vi "Teleop.vi"(10 "Match Info":T1={"Autonomous Elapsed Seconds"=0.0, "TeleOp Elapsed Seconds"=0.0, "Disabled Elapsed Seconds"=0.0, "Visited Autonomous"=FALSE, "Visited TeleOp"=FALSE, "Visited Disabled"=FALSE, "Autonomous Settings"={"Autonomous Style"=enum."Independent", "VI Refnum"=refnum}}, 11 "Call Context":T2) -> ()   [LabVIEW 2014]
doc: "This VI is called for each TeleOp packet received from the DS where the robot is not disabled. It is often used to read from the joysticks and update I/O or to update setpoints for timed control loops. It should complete and return within 20 milliseconds or it may miss DS packets."
uses:
  Robot Global Data.vi
  <vilib>/functionblocks/FB Core/FB Core.xnode
  <vilib>/functionblocks/Edge Detection/Edge Detect/Edge Detect.vi
  <vilib>/functionblocks/NI_FunctionBlock Libraries.lvlib
  <vilib>/Rock Robotics/WPI/Relay/WPI_RelayValue.ctl
  <vilib>/Rock Robotics/WPI/RobotDrive/WPI_RobotDriveMecanumDrive_Cartesian.vi
  <vilib>/Rock Robotics/WPI/DriverStation/WPI_DriverStationMatch Info.ctl
  <vilib>/Rock Robotics/WPI/DriverStation/WPI_DriverStationDerivedRobotMode.ctl
panel:
  out "One Driver":bool
  out "Loader Up":bool
  out "Right Bumper":bool
  out "Left Bumper":bool
  out "Loader Out":bool
  out "Ejector":bool
  out "Trigger":bool
  out "1 Cylinder":bool
  out "2 Cylinder":bool
  out "3 Cylinder":bool
  out "Motor Values":dbl[](array[numeric])
  out "Gyro Mode?":bool
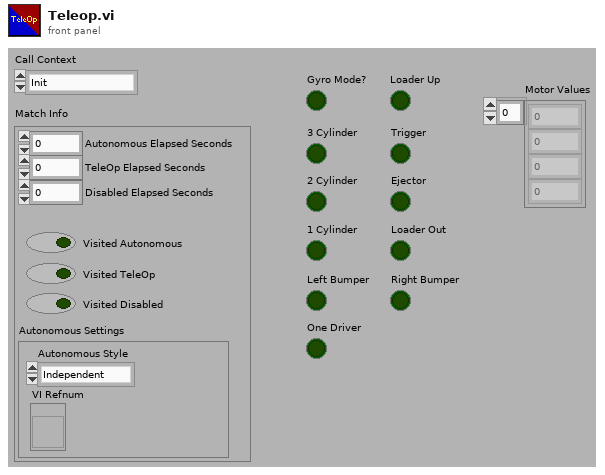
[diagram p1: front panel]
types:
  T1 = typedef "WPI_DriverStationMatch Info.ctl" = cluster{"Autonomous Elapsed Seconds":dbl, "TeleOp Elapsed Seconds":dbl, "Disabled Elapsed Seconds":dbl, "Visited Autonomous":bool, "Visited TeleOp":bool, "Visited Disabled":bool, "Autonomous Settings":cluster{"Autonomous Style":enum16{"Iterative", "Independent"}, "VI Refnum":refnum<vi>}}
  T2 = typedef "WPI_DriverStationDerivedRobotMode.ctl" = enum16{"Init", "Execute", "Stop"}
  T3 = typedef "WPI_RelayValue.ctl" = enum16{"Off", "On", "Forward", "Reverse"}
  T4 = typedef "WPI_JoystickDevRef.ctl" = cluster{"Device":T5}
  T5 = typedef "WPI_JoystickDeviceEnum.ctl" = enum16{"USB 1", "USB 2", "USB 3", "USB 4", "Kinect 1", "Kinect 2"}
  T6 = typedef "WPI_JoystickButtonState.ctl" = cluster{"Button 1":bool, "Button 2":bool, "Button 3":bool, "Button 4":bool, "Button 5":bool, "Button 6":bool, "Button 7":bool, "Button 8":bool, "Button 9":bool, "Button 10":bool, "Button 11":bool, "Button 12":bool}
  T7 = cluster{"axis 1 (x)":dbl, "axis 2 (y)":dbl, "axis 3 (throttle)":dbl, "axis 4":dbl, "axis 5":dbl, "axis 6":dbl}
  T8 = typedef "WPI_DigitalInputDevRef.ctl" = cluster{"DevStatus":errorcluster, "DIO Channel":T9, "Digital Module":T10}
  T9 = typedef "FPGA_DIOChannel.ctl" = enum8{"DIO 1", "DIO 2", "DIO 3", "DIO 4", "DIO 5", "DIO 6", "DIO 7", "DIO 8", "DIO 9", "DIO 10", "DIO 11", "DIO 12", "DIO 13", "DIO 14", "Invalid"}
  T10 = typedef "FPGA_TypedefDigitalModule.ctl" = enum16{"Digital Module 1", "Digital Module 2"}
  T11 = typedef "WPI_MotorControlDeviceRef.ctl" = cluster{"DeviceStatus":errorcluster, "Type":enum16{"PWM", "CAN"}, "PWM":cluster{"Digital Module":T10, "PWM Channel":T12, "DeadBand":T13}, "CAN":cluster{"Device Number":u8, "Control Mode":T14, "Semaphore":T15, "Max Vout":dbl}, "Invert":bool, "TransformRef":T16, "InvTransformRef":T16}
  T12 = typedef "FPGA_DIOPWMChannel.ctl" = enum8{"PWM 1", "PWM 2", "PWM 3", "PWM 4", "PWM 5", "PWM 6", "PWM 7", "PWM 8", "PWM 9", "PWM 10", "Invalid"}
  T13 = typedef "WPI_PWMDeadband.ctl" = cluster{"Name":string, "maxPositivePwm":i32, "minPositivePwm":i32, "centerPwm":i32, "maxNegativePwm":i32, "minNegativePwm":i32, "angularRange":u16}
  T14 = typedef "WPI_CANJaguar_ControlMode.ctl" = enum8{"Percent VBus", "Current", "Speed", "Position", "Voltage"}
  T15 = typedef "Semaphore RefNum" = refnum<k1>
  T16 = typedef "WPI_PWMTransform_ConPane.ctl" = refnum<vi>
  T17 = typedef "WPI_RelayDevRef.ctl" = cluster{"DevStatus":errorcluster, "Relay Channel":T18, "Digital Module":T10, "Relay Direction":T19}
  T18 = typedef "FPGA_DIORelayChannel.ctl" = enum8{"Relay 1", "Relay 2", "Relay 3", "Relay 4", "Relay 5", "Relay 6", "Relay 7", "Relay 8", "Invalid"}
  T19 = typedef "WPI_RelayDirection.ctl" = enum16{"Both directions", "Forward only", "Reverse only"}
  T20 = typedef "WPI_RobotDriveDevRef.ctl" = cluster{"DevStatus":errorcluster, "Motors[]":T11[], "Square Inputs":bool, "Max Output":dbl, "Isochronous":bool}
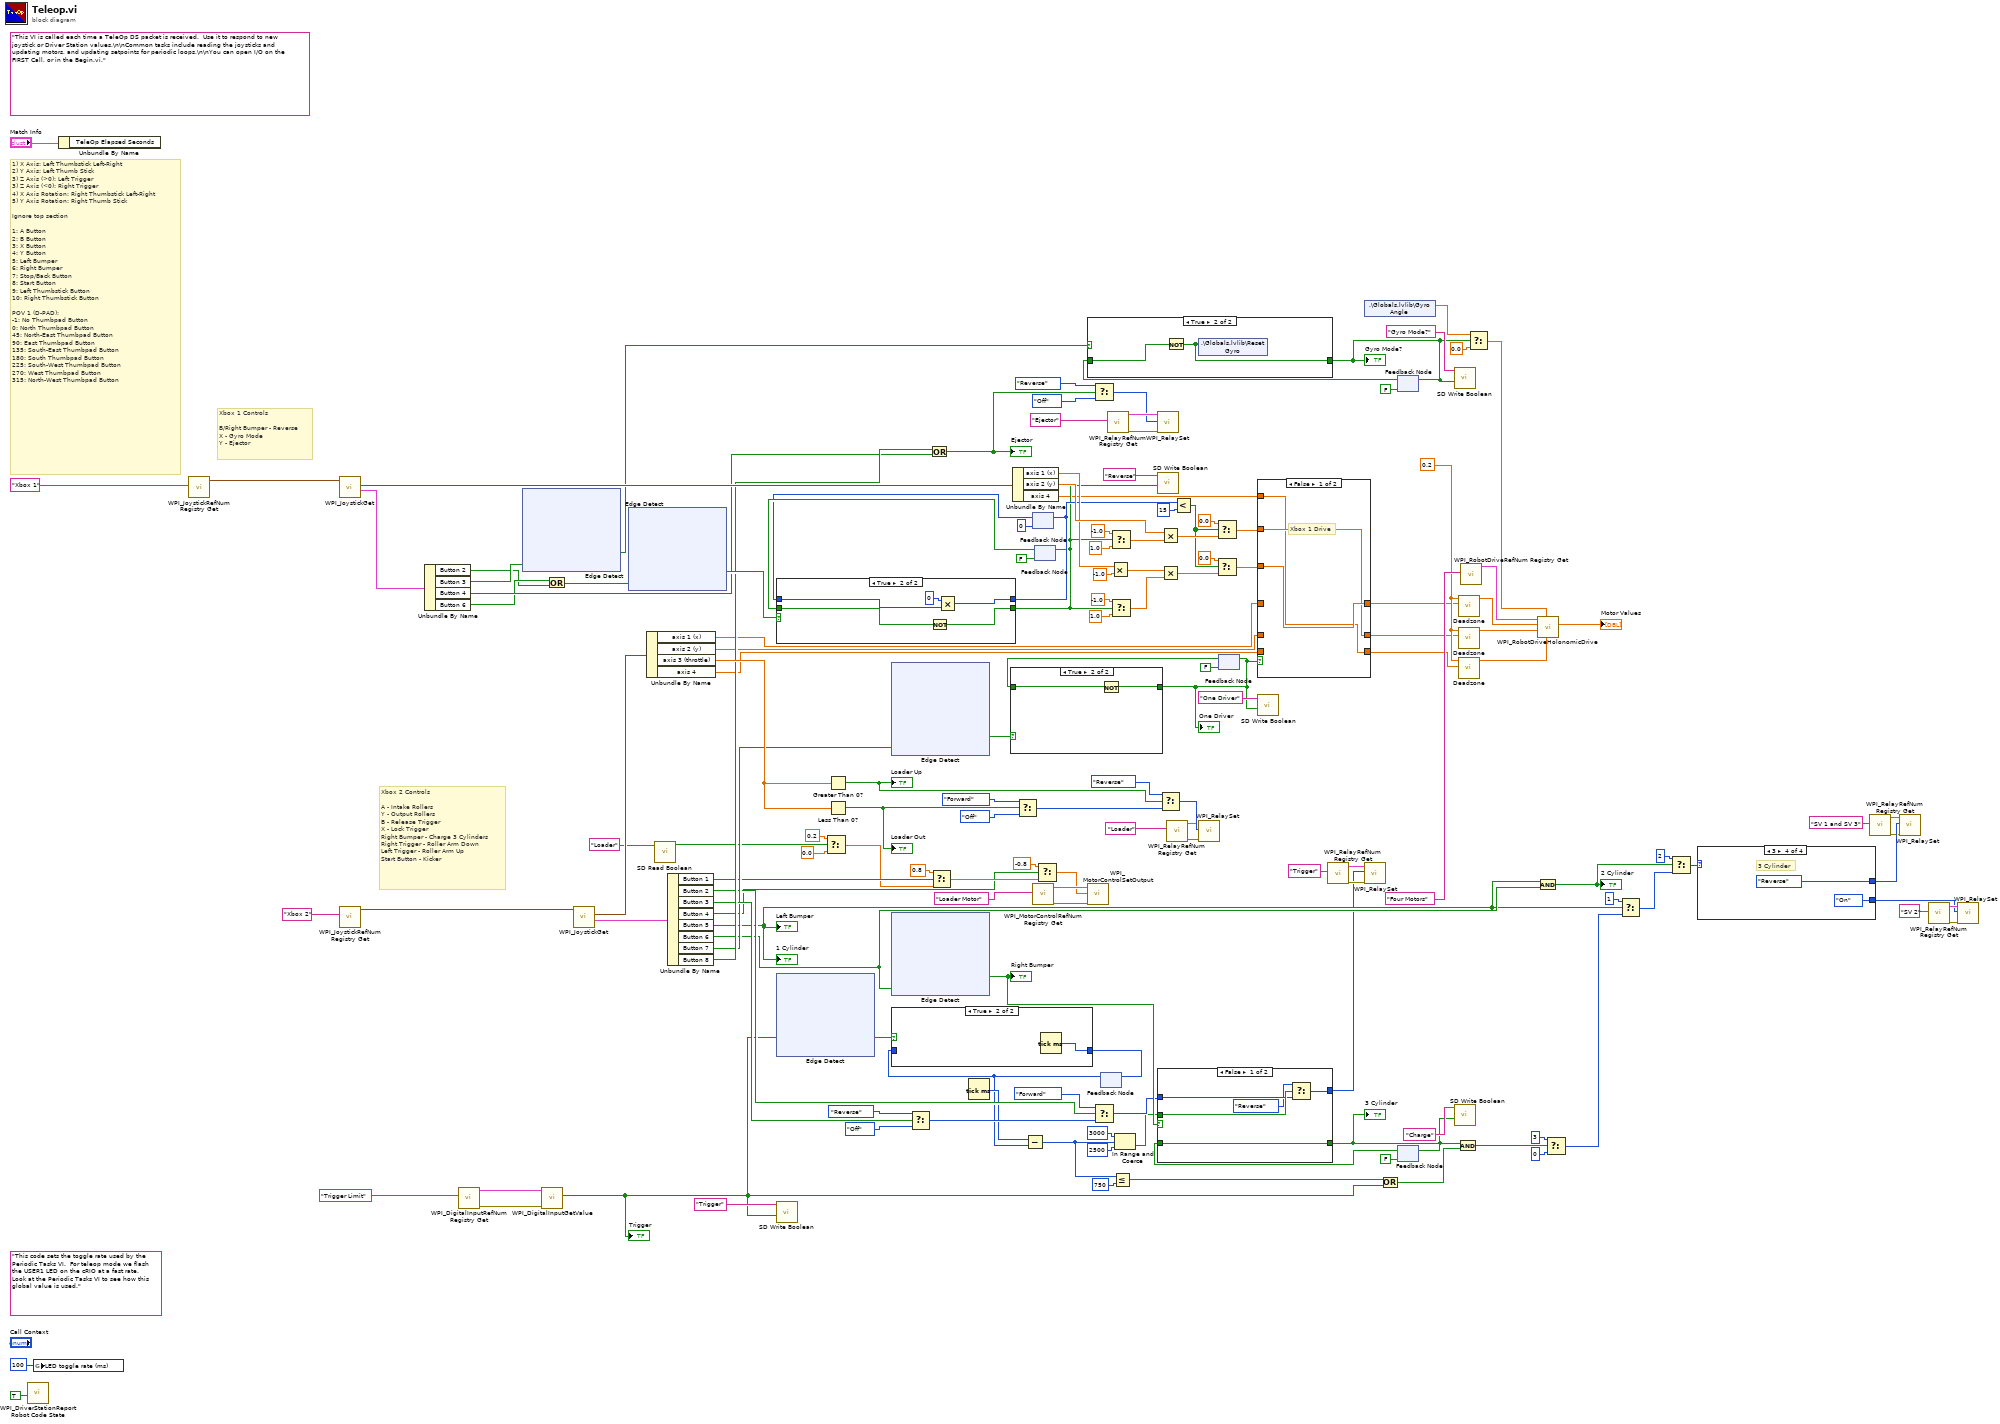
[diagram p0: block diagram]
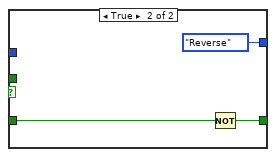
[diagram p3: hidden frame]
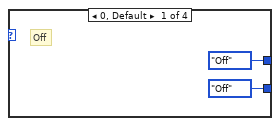
[diagram p6: hidden frame]
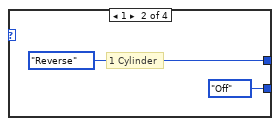
[diagram p7: hidden frame]
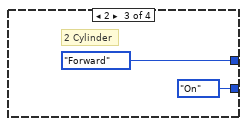
[diagram p8: hidden frame]
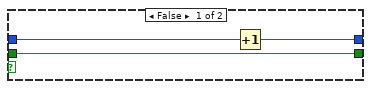
[diagram p9: hidden frame]
diagram:
  w56 = 0.2 ("Deadzone")
  (unwired) "This code sets the toggle rate used by the Periodic Tasks VI.  For teleop mode we flash the USER1 LED on the cRIO at a fast rate.  Look at the Periodic Tasks VI to see how this global value is used."
  (unwired) "This VI is called each time a TeleOp DS packet is received.  Use it to respond to new joystick or Driver Station values.\n\nCommon tasks include reading the joysticks and updating motors, and updating setpoints for periodic loops.\n\nYou can open I/O on the FIRST Call, or in the Begin.vi."
  # "Xbox 1 Controls\n\nB/Right Bumper - Reverse\nX - Gyro Mode\nY - Ejector"
  # "Xbox 2 Controls\n\nA - Intake Rollers\nY - Output Rollers\nB - Release Trigger\nX - Lock Trigger\nRight Bumper - Charge 3 Cylinders\nRight Trigger - Roller Arm Down\nLeft Trigger - Roller Arm Up\nStart Button - Kicker"
  # "1) X Axis: Left Thumbstick Left-Right\n2) Y Axis: Left Thumb Stick\n3) Z Axis (>0): Left Trigger\n3) Z Axis (<0): Right Trigger\n4) X Axis Rotation: Right Thumbstick Left-Right\n5) Y Axis Rotation: Right Thumb Stick\n\nIgnore top section\n\n1: A Button\n2: B Button\n3: X Button\n4: Y Button\n5: Left Bumper\n6: Right Bumper\n7: Stop/Back Button\n8: Start Button\n9: Left Thumbstick Button\n10: Right Thumbstick Button\n\nPOV 1 (D-PAD):\n-1: No Thumbpad Button\n0: North Thumbpad Button\n45: North-East Thumbpad Button\n90: East Thumbpad Button\n135: South-East Thumbpad Button\n180: South Thumbpad Button\n225: South-West Thumbpad Button\n270: West Thumbpad Button\n315: North-West Thumbpad Button"
  n1 = call <vilib>:"WPI_DriverStationReport Robot Code State.vi"("TeleOp"=TRUE ("Autonomous")) -> ()  [unwired: 10 in, 1 out]
  n2 = global write "Robot Global Data.vi" "LED toggle rate (ms)"(u32 100 ("LED ms toggle rate")) -> ()
  n3 = Unbundle By Name("Match Info") -> ()  [unwired: 1 out]
  n4 = call <vilib>:"WPI_JoystickRefNum Registry Get.vi"("refnum name"="Xbox 1") -> ("JoystickDevRef"=w152:T4)  [unwired: 1 in, 9 out]
  n5 = call <vilib>:"WPI_JoystickGet.vi"("JoystickDevRef"=w152) -> ("Buttons"=w144:T6, "Axes"=w149:T7)  [unwired: 1 in, 4 out]
  n6 = call <vilib>:"WPI_JoystickRefNum Registry Get.vi"("refnum name"="Xbox 2") -> ("JoystickDevRef"=w123:T4)  [unwired: 1 in, 9 out]
  n7 = Unbundle By Name(w144) -> ("Button 2"=w58:bool, "Button 3"=w77:bool, "Button 4"=w65:bool, "Button 6"=w59:bool)
  n8 = call <vilib>:"WPI_DigitalInputRefNum Registry Get.vi"("refnum name"="Trigger Limit") -> ("error out"=w32:errorcluster, "DigitalInputDevRef"=w31:T8)  [unwired: 9 in]
  n9 = xnode "Edge Detect"("input 1"=w77) -> ("output"=w81:bool)  [unwired: 2 in, 1 out]
  n10 = call <vilib>:"WPI_DigitalInputGetValue.vi"("error in (no error)"=w32, "DigitalInputDevRef"=w31) -> ("Value"=w16:bool)  [unwired: 7 in, 2 out]
  "Trigger" <- w16
  n11 = Or(x=w59, y=w58) -> (x .or. y?=w57:bool)
  n12 = call <vilib>:"WPI_JoystickGet.vi"("JoystickDevRef"=w123) -> ("Buttons"=w121:T6, "Axes"=w120:T7)  [unwired: 1 in, 4 out]
  n13 = xnode "Edge Detect"("input 1"=w57) -> ("output"=w131:bool)  [unwired: 2 in, 1 out]
  n14 = Unbundle By Name(w120) -> ("axis 1 (x)"=w48:dbl, "axis 2 (y)"=w47:dbl, "axis 3 (throttle)"=w76:dbl, "axis 4"=w46:dbl)
  n15 = call <vilib>:"SD Read Boolean.vi"("Name"="Loader") -> ("Boolean"=w4:bool)  [unwired: 8 in, 2 out]
  n16 = Unbundle By Name(w121) -> ("Button 1"=w38:bool, "Button 2"=w39:bool, "Button 3"=w64:bool, "Button 4"=w37:bool, "Button 5"=w29:bool, "Button 6"=w30:bool, "Button 7"=w45:bool, "Button 8"=w67:bool)
  "1 Cylinder" <- w29
  "Left Bumper" <- w29
  n17 = xnode "Edge Detect"("input 2"=w16) -> ("output"=w22:bool)  [unwired: 2 in, 1 out]
  n18 = call <vilib>:"SD Write Boolean.vi"("Boolean"=w16, "Name"="Trigger") -> ()  [unwired: 8 in, 2 out]
  n19 = Select(t=0.2 ("idle speed"), s=w4, f=0.0) -> (s? t:f=w1:dbl)
  n20 = Greater Than 0?(x=w76) -> (x > 0?=w10:bool)
  "Loader Up" <- w10
  n21 = Less Than 0?(x=w76) -> (x < 0?=w11:bool)
  "Loader Out" <- w11
  n22 = xnode "Edge Detect"("input 1"=w45) -> ("output"=w42:bool)  [unwired: 2 in, 1 out]
  n23 = xnode "Edge Detect"("input 1"=w30) -> ("output"=w35:bool)  [unwired: 2 in, 1 out]
  "Right Bumper" <- w35
  n24 = Select(t=WPI_RelayValue."Reverse" ("RelayValue"), s=w64, f=WPI_RelayValue."Off") -> (s? t:f=w107:T3)
  n25 = Or(x=w67, y=w65) -> (x .or. y?=w66:bool)
  "Ejector" <- w66
  n26 = Select(t=0.8, s=w38, f=w1) -> (s? t:f=w84:dbl)
  n27 = Tick Count (ms)() -> (millisecond timer value=w20:u32)
  n28 = Unbundle By Name(w149) -> ("axis 1 (x)"=w146:dbl, "axis 2 (y)"=w147:dbl, "axis 4"=w50:dbl)
  n29 = Select(t=WPI_RelayValue."Forward" ("RelayValue"), s=w11, f=WPI_RelayValue."Off") -> (s? t:f=w103:T3)
  n30 = feedback #1(0) -> (w126:i32)
  n31 = call <vilib>:"WPI_MotorControlRefNum Registry Get.vi"("refnum name"="Loader Motor") -> ("error out"=w85:errorcluster, "MotorControlDevRef"=w86:T11)  [unwired: 9 in]
  n32 = feedback #2(FALSE) -> (w133:bool)
  n33 = case shown="True" w131 {
    tunnel: w133 -> [w157 w162]
    tunnel: [w157 w161] -> w69
    tunnel: w126 -> [w156 w160]
    tunnel: [w155 w158] -> w125
    frame False {
      n34 = Increment(x=w156) -> (x+1=w155:i32)
    }
    frame True {
      n35 = Not(x=w162) -> (.not. x?=w161:bool)
      n36 = Multiply(x=0, y=w160) -> (x*y=w158:i32)
    }
  }
  n37 = feedback-in #1(w125) -> ()
  n38 = feedback-in #2(w69) -> ()
  n39 = Select(t=-0.8, s=w37, f=w84) -> (s? t:f=w55:dbl)
  n40 = call <vilib>:"WPI_MotorControlSetOutput.vi"("error in (no error)"=w85, "Output"=w55, "MotorControlDevRef"=w86) -> ()  [unwired: 6 in, 3 out]
  n41 = Select(t=WPI_RelayValue."Reverse" ("f"), s=w66, f=WPI_RelayValue."Off") -> (s? t:f=w89:T3)
  n42 = Select(t=WPI_RelayValue."Forward" ("RelayValue"), s=w39, f=w107) -> (s? t:f=w24:T3)
  n43 = feedback #3() -> (w19:u32)  [unwired: 1 in]
  n44 = case shown="True" w22 {
    tunnel: [w163 w164] -> w21
    tunnel: w19 -> [w163 _]
    frame False {
    }
    frame True {
      n45 = Tick Count (ms)() -> (millisecond timer value=w164:u32)
    }
  }
  n46 = Subtract(x=w20, y=w19) -> (x-y=w9:u32)
  n47 = feedback-in #3(w21) -> ()
  n48 = call <vilib>:"WPI_RelayRefNum Registry Get.vi"("refnum name"="Ejector") -> ("error out"=w94:errorcluster, "RelayDevRef"=w92:T17)  [unwired: 9 in]
  n49 = Multiply(x=w146, y=-1.0) -> (x*y=w68:dbl)
  n50 = Select(t=-1.0, s=w69, f=1.0) -> (s? t:f=w136:dbl)
  n51 = Select(t=-1.0, s=w69, f=1.0) -> (s? t:f=w72:dbl)
  n52 = Less Or Equal?(x=w9, y=u32 750) -> (x <= y?=w17:bool)
  n53 = In Range and Coerce(upper limit=u32 3000 ("y"), x=w9, lower limit=u32 2500 ("y")) -> (In Range?=w6:bool)  [unwired: 1 out]
  n54 = call <vilib>:"WPI_RelaySet.vi"("error in (no error)"=w94, "RelayValue"=w89, "RelayDevRef"=w92) -> ()  [unwired: 7 in, 2 out]
  n55 = call <vilib>:"SD Write Boolean.vi"("Boolean"=w69, "Name"="Reverse") -> ()  [unwired: 8 in, 2 out]
  n56 = Multiply(x=w147, y=w136) -> (x*y=w129:dbl)
  n57 = Multiply(x=w68, y=w72) -> (x*y=w73:dbl)
  n58 = Select(t=WPI_RelayValue."Reverse" ("RelayValue"), s=w10, f=w103) -> (s? t:f=w104:T3)
  n59 = call <vilib>:"WPI_RelayRefNum Registry Get.vi"("refnum name"="Loader") -> ("error out"=w98:errorcluster, "RelayDevRef"=w99:T17)  [unwired: 9 in]
  n60 = Less?(x=w125, y=15) -> (x < y?=w74:bool)
  n61 = call <vilib>:"WPI_RelaySet.vi"("error in (no error)"=w98, "RelayValue"=w104, "RelayDevRef"=w99) -> ()  [unwired: 7 in, 2 out]
  n62 = Select(t=0.0, s=w74, f=w129) -> (s? t:f=w52:dbl)
  n63 = Select(t=0.0, s=w74, f=w73) -> (s? t:f=w54:dbl)
  n64 = feedback #4(FALSE) -> (w41:bool)
  n65 = case shown="True" w42 {
    tunnel: [w165 w167] -> w40
    tunnel: w41 -> [w165 w166]
    frame False {
    }
    frame True {
      n66 = Not(x=w166) -> (.not. x?=w167:bool)
    }
  }
  "One Driver" <- w40
  n67 = feedback-in #4(w40) -> ()
  n68 = case shown="False" w40 {
    tunnel: w54 -> [w170 _]
    tunnel: [w170 w173] -> w53
    tunnel: w52 -> [w169 _]
    tunnel: [w169 w172] -> w51
    tunnel: w50 -> [w168 _]
    tunnel: [w168 w171] -> w49
    tunnel: w48 -> [_ w173]
    tunnel: w47 -> [_ w172]
    tunnel: w46 -> [_ w171]
    frame False {
      # "Xbox 1 Drive"
    }
    frame True {
      # "Xbox 2 Drive"
    }
  }
  n69 = call <vilib>:"SD Write Boolean.vi"("Boolean"=w40, "Name"="One Driver") -> ()  [unwired: 8 in, 2 out]
  n70 = call <vilib>:"WPI_RelayRefNum Registry Get.vi"("refnum name"="Trigger") -> ("error out"=w97:errorcluster, "RelayDevRef"=w111:T17)  [unwired: 9 in]
  n71 = shared-variable ".\\Globals.lvlib\\Gyro Angle"() -> (w143:dbl)  [unwired: 1 in, 1 out]
  n72 = Or(x=w17, y=w16) -> (x .or. y?=w15:bool)
  n73 = feedback #5(FALSE) -> (w140:bool)
  n74 = case shown="True" w81 {
    tunnel: w140 -> [w174 w176]
    tunnel: [w174 w175] -> w25
    frame False {
    }
    frame True {
      n75 = Not(x=w176) -> (.not. x?=w175:bool)
      n76 = shared-variable ".\\Globals.lvlib\\Reset Gyro"(w175) -> ()  [unwired: 1 in, 1 out]
    }
  }
  "Gyro Mode?" <- w25
  n77 = feedback-in #5(w25) -> ()
  n78 = feedback #6(FALSE) -> (w34:bool)
  n79 = case shown="False" w35 {
    tunnel: w34 -> [w181 w184]
    tunnel: [w181 w183] -> w12
    tunnel: w24 -> [w179 _]
    tunnel: [w178 WPI_RelayValue."Reverse" ("f")] -> w23
    tunnel: w6 -> [w180 _]
    frame False {
      n80 = Select(t=WPI_RelayValue."Reverse", s=w180, f=w179) -> (s? t:f=w178:T3)
    }
    frame True {
      n81 = Not(x=w184) -> (.not. x?=w183:bool)
    }
  }
  "3 Cylinder" <- w12
  n82 = call <vilib>:"WPI_RelaySet.vi"("error in (no error)"=w97, "RelayValue"=w23, "RelayDevRef"=w111) -> ()  [unwired: 7 in, 2 out]
  n83 = feedback-in #6(w12) -> ()
  n84 = call <vilib>:"SD Write Boolean.vi"("Boolean"=w25, "Name"="Gyro Mode?") -> ()  [unwired: 8 in, 2 out]
  n85 = call <vilib>:"SD Write Boolean.vi"("Boolean"=w12, "Name"="Charge") -> ()  [unwired: 8 in, 2 out]
  n86 = And(x=w12, y=w15) -> (x .and. y?=w13:bool)
  n87 = call "Deadzone.vi"("Input"=w53, "Deadzone"=w56) -> ("Corected"=w61:dbl)  [unwired: 9 in]
  n88 = call "Deadzone.vi"("Input"=w51, "Deadzone"=w56) -> ("Corected"=w60:dbl)  [unwired: 9 in]
  n89 = call "Deadzone.vi"("Input"=w49, "Deadzone"=w56) -> ("Corected"=w62:dbl)  [unwired: 9 in]
  n90 = call <vilib>:"WPI_RobotDriveRefNum Registry Get.vi"("refnum name"="Four Motors") -> ("RobotDriveDevRef"=w80:T20)  [unwired: 1 in, 9 out]
  n91 = Select(t=w143, s=w25, f=0.0) -> (s? t:f=w78:dbl)
  n92 = call-poly <vilib>:"WPI_RobotDriveHolonomicDrive.vi"("Rotation"=w62, "Gyro Angle"=w78, "Y"=w60, "X"=w61, "RobotDriveDevRef"=w80) -> ("Motor Values"=→"Motor Values":dbl[])  [unwired: 4 in, 2 out]
  n93 = And(x=w29, y=w30) -> (x .and. y?=w88:bool)
  "2 Cylinder" <- w88
  n94 = Select(t=3, s=w13, f=0) -> (s? t:f=w28:i32)
  n95 = Select(t=1, s=w29, f=w28) -> (s? t:f=w27:i32)
  n96 = Select(t=2, s=w88, f=w27) -> (s? t:f=w26:i32)
  n97 = case shown="3" w26 {
    tunnel: [WPI_RelayValue."Off" ("RelayValue") WPI_RelayValue."Reverse" ("RelayValue") WPI_RelayValue."Forward" ("RelayValue") WPI_RelayValue."Reverse" ("RelayValue")] -> w113
    tunnel: [WPI_RelayValue."Off" ("RelayValue") WPI_RelayValue."Off" ("RelayValue") WPI_RelayValue."On" ("RelayValue") WPI_RelayValue."On" ("RelayValue")] -> w112
    frame 0, Default {
      # "Off"
    }
    frame 1 {
      # "1 Cylinder"
    }
    frame 2 {
      # "2 Cylinder"
    }
    frame 3 {
      # "3 Cylinder"
    }
  }
  n98 = call <vilib>:"WPI_RelayRefNum Registry Get.vi"("refnum name"="SV 1 and SV 3") -> ("error out"=w95:errorcluster, "RelayDevRef"=w137:T17)  [unwired: 9 in]
  n99 = call <vilib>:"WPI_RelaySet.vi"("error in (no error)"=w95, "RelayValue"=w113, "RelayDevRef"=w137) -> ()  [unwired: 7 in, 2 out]
  n100 = call <vilib>:"WPI_RelayRefNum Registry Get.vi"("refnum name"="SV 2") -> ("error out"=w96:errorcluster, "RelayDevRef"=w118:T17)  [unwired: 9 in]
  n101 = call <vilib>:"WPI_RelaySet.vi"("error in (no error)"=w96, "RelayValue"=w112, "RelayDevRef"=w118) -> ()  [unwired: 7 in, 2 out]
